vi "Solve General Linear Equations.vi"(2 "relative tolerance":dbl, 3 "Known Vector":dbl[](array[numeric]) format="%.2f", 4 "Input Matrix":T1) -> (0 "error":i32, 1 "Solution Vector":dbl[](array[numeric]) format="%.2f")   [LabVIEW 2010, in "NI_AALBase.lvlib"]
doc: "Solves a real linear system AX=Y using svd algorithm.\n If A is full rank, the vi finds the solution. In the case of multiple solutions, it finds the minimum 2-norm solution.\n If A is rank deficit, the vi finds the least square solution.\n\nInput Matrix is a square or rectangular, real matrix.\nKnown Vector. The number of elements in the Known Vector must be equal to the rows of the Input Matrix. If the number of elements in the Known Vector does not match the rows of the Input Matrix, the VI sets the Solution Vector to an empty array and returns an error.\n\nSolution Vector is the solution X to AX = Y.\n\nLet A be an m-by-n matrix that represents the Input Matrix, Y be the set of m coefficients in Known Vector, and X be the set of n elements in Solution Vector that solves the system AX = Y."
uses:
  NI_AALBase.lvlib
  RealMatrix.ctl
  lvanlys.dll
  NI_Matrix.lvlib
panel:
  # "Solve General Linear Equations"
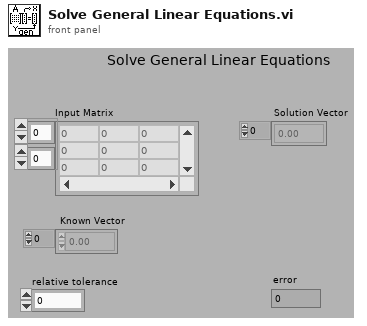
[diagram p1: front panel]
types:
  T1 = typedef "NI_Matrix.lvlib/RealMatrix.ctl" = dbl[][]
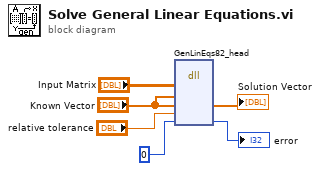
[diagram p0: block diagram]
diagram:
  n1 = dll-call lib="C:/Program Files/National Instruments/LabVIEW 2010/resource/lvanlys.*" fn="GenLinEqs82_head"("aH"="Input Matrix", "bH"="Known Vector", "xH"="Known Vector", "relativeTol"="relative tolerance", "dsperr"=0) -> ("xH"=→"Solution Vector":dbl[], "dsperr"=→"error":i32)  [unwired: 7 in, 2 out]
